vi "niRFUtil TRC Waveform to Trace (complex array).vi"(7 "Complex Array":T2 format="%.2f") -> (8 "Measurement Trace":T1 format="%.2f")   [LabVIEW 2015, in "niRFUtil.lvlib"]
doc: "(c) Copyright 2006, National Instruments, Inc. This VI may not be duplicated, sold, or distributed without written consent from National Instruments."
uses:
  niRFUtil.lvlib
  Includes/niRFUtil INC Complex Array.ctl
  Includes/niRFUtil INC Trace.ctl
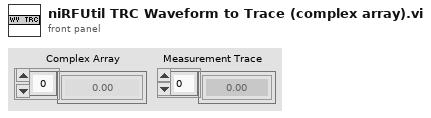
[diagram p1: front panel]
types:
  T1 = typedef "niRFUtil.lvlib/niRFUtil INC Trace.ctl" = sgl[]
  T2 = typedef "niRFUtil.lvlib/niRFUtil INC Complex Array.ctl" = csg[]
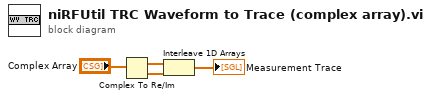
[diagram p0: block diagram]
diagram:
  n1 = Complex To Re/Im(x + iy="Complex Array") -> (x=w3:sgl[], y=w4:sgl[])
  n2 = Interleave 1D Arrays(w3, w4) -> (→"Measurement Trace":sgl[])
